vi "ALL Loop Status.vi"(6 "Status List":bool[](array[boolean])=[FALSE, FALSE, FALSE, FALSE, FALSE, FALSE, FALSE, FALSE], 7 "Option":T2(ring), 8 "error in (no error)":errorcluster, 9 "Status":bool, 10 "Loops":T1[](array[typedef]), 11 "Loop":T1) -> (0 "error out":errorcluster, 2 "Status Out":bool, 3 "Status List Out":bool[](array[boolean]))   [LabVIEW 2022 SP3]
uses:
  Controls/All Loop Status.ctl
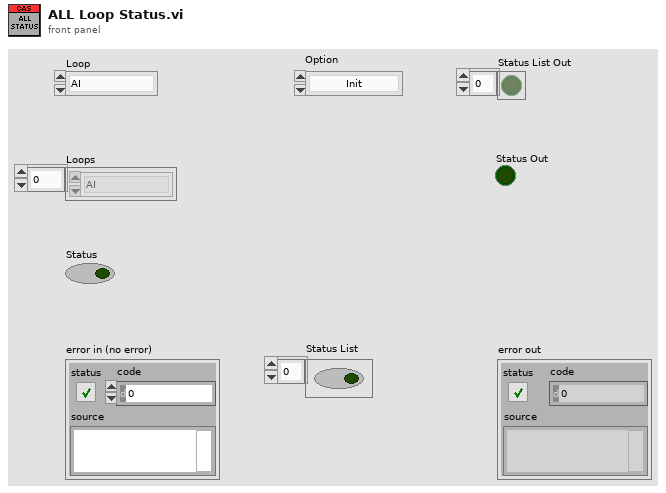
[diagram p1: front panel]
types:
  T1 = typedef "All Loop Status.ctl" = enum16{"AI", "AO", "DI", "DO", "TC", "Strain", "ACC", "RT", "Log"}
  T2 = enum16{"Init", "Read 'All'", "Read 'n'", "Read '1'", "Write '1'", "Write 'n'", "Write 'All'"}
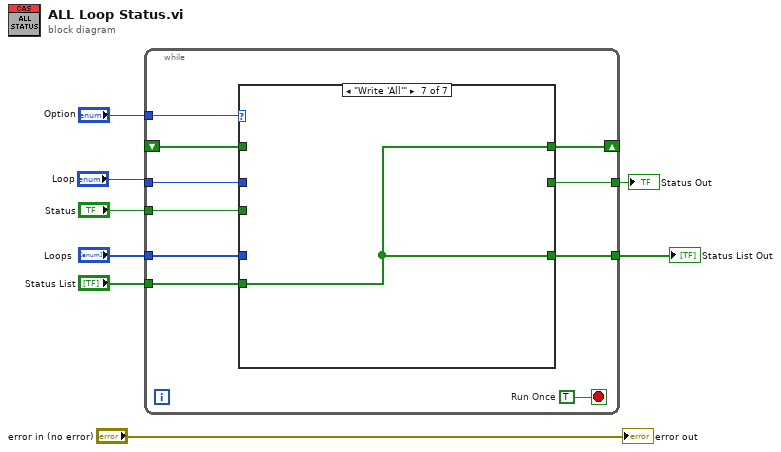
[diagram p0: block diagram]
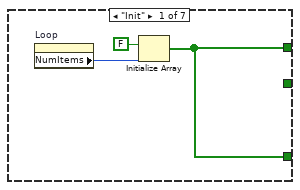
[diagram p2: hidden frame]
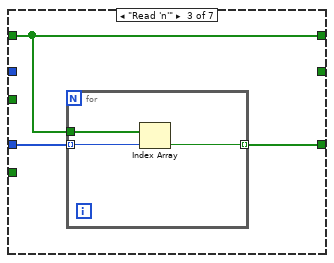
[diagram p4: hidden frame]
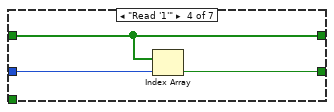
[diagram p5: hidden frame]
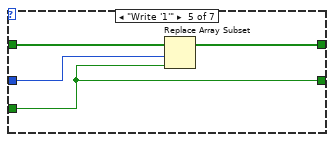
[diagram p6: hidden frame]
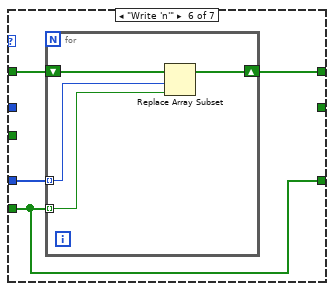
[diagram p7: hidden frame]
diagram:
  n1 = while {
    tunnel: "Option" -> [w17]
    shift-right: [w16] -> _
    shift-left: _ -> [w15]
    tunnel: "Loops" -> [w14]
    tunnel: [w13] -> w6
    tunnel: "Loop" -> [w12]
    tunnel: [w11] -> w5
    tunnel: "Status" -> [w10]
    tunnel: "Status List" -> [w9]
    stop <- w18 stop-if-true
    w18 = TRUE  # Run Once
    n2 = case shown="\"Write 'All'\"" w17 {
      tunnel: [w20 w22 w24 w31 w34 w38 w44] -> w16
      tunnel: w15 -> [_ w22 w24 w31 w35 w39 _]
      tunnel: w14 -> [_ _ w25 _ _ w37 _]
      tunnel: [w20 w22 w23 _ _ w36 w44] -> w13
      tunnel: w12 -> [_ _ _ w30 w33 _ _]
      tunnel: [_ _ _ w29 w32 _ _] -> w11
      tunnel: w10 -> [_ _ _ _ w32 _ _]
      tunnel: w9 -> [_ _ _ _ _ w36 w44]
      frame "Init" {
        n3 = property on="Loop" class="Enum (strict)"() -> ("NumItems"=w19:u32)  [unwired: 2 in, 2 out]
        n4 = Initialize Array(FALSE, w19) -> (w20:bool[])
      }
      frame "Read 'All'", Default {
      }
      frame "Read 'n'" {
        n5 = for {
          tunnel: w25 -> [w27] mode=indexing
          tunnel: w24 -> [w28]
          tunnel: [w26] -> w23 mode=indexing
          n6 = Index Array(array=w28, index=w27) -> (element=w26:bool)
        }
      }
      frame "Read '1'" {
        n7 = Index Array(array=w31, index=w30) -> (element=w29:bool)
      }
      frame "Write '1'" {
        n8 = Replace Array Subset(array=w35, new element=w32, index=w33) -> (w34:bool[])
      }
      frame "Write 'n'" {
        n9 = for {
          tunnel: w37 -> [w41] mode=indexing
          tunnel: w36 -> [w40] mode=indexing
          shift-right: [w42] -> w38
          shift-left: w39 -> [w43]
          n10 = Replace Array Subset(array=w43, new element=w40, index=w41) -> (w42:bool[])
        }
      }
      frame "Write 'All'" {
      }
    }
  }
  "Status List Out" <- w6
  "Status Out" <- w5
  "error out" <- "error in (no error)"
